vi "Calc Max During Mem Fill 2.vi"(7 "Value":fxp<+/-,22,22>, 8 "LastIterration":bool, 9 "ActiveLedIndex":u32, 10 "FirstIterration":bool, 11 "Address":u32) -> ()   [LabVIEW 2013]
uses:
  <vilib>/rvi/Emulation/niFpgaSctlEmulationGetInTimedLoop.vi
  LIDAR V2 Globals.vi
  <vilib>/rvi/Emulation/niFpgaProcessEmulError.vi
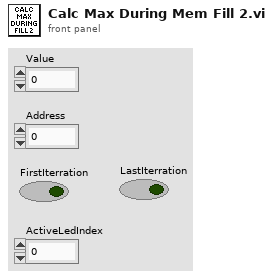
[diagram p1: front panel]
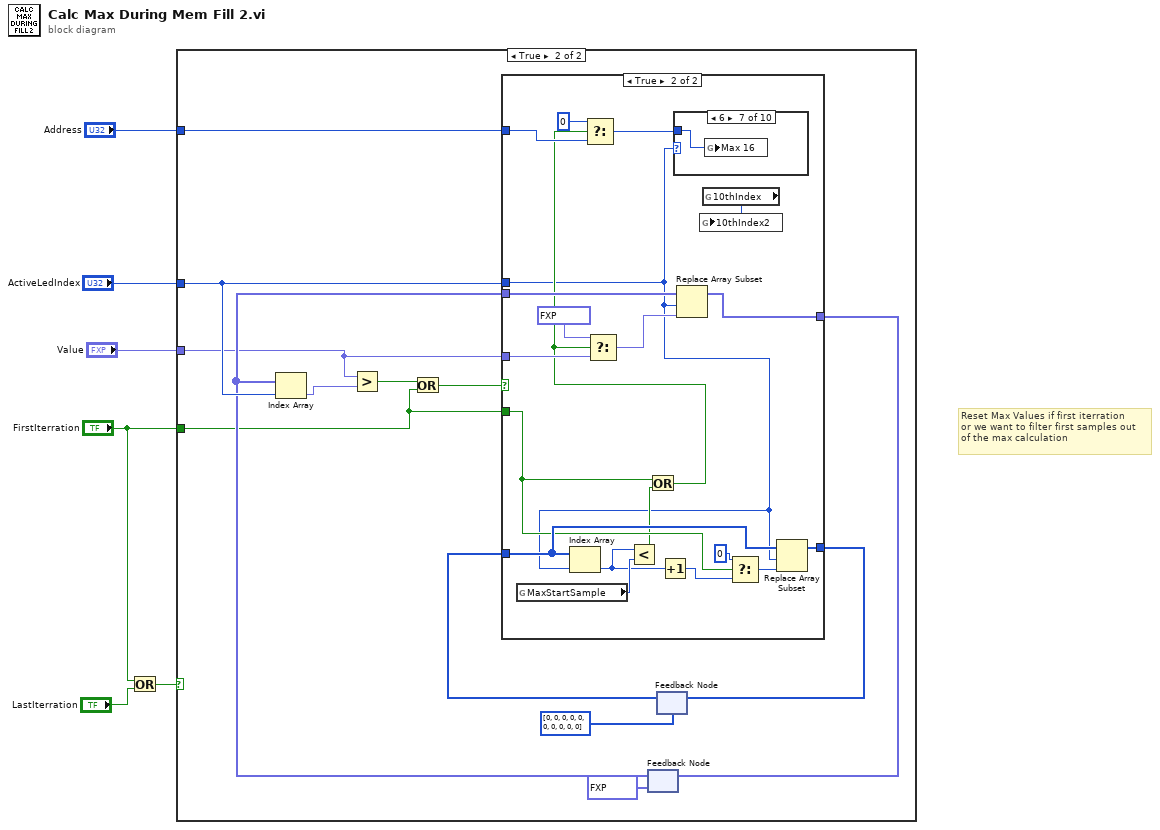
[diagram p0: block diagram]
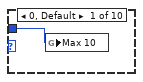
[diagram p4: hidden frame]
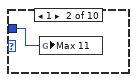
[diagram p5: hidden frame]
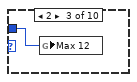
[diagram p6: hidden frame]
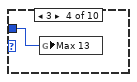
[diagram p7: hidden frame]
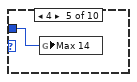
[diagram p8: hidden frame]
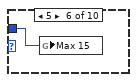
[diagram p9: hidden frame]
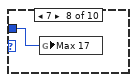
[diagram p10: hidden frame]
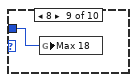
[diagram p11: hidden frame]
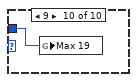
[diagram p12: hidden frame]
diagram:
  # "Reset Max Values if first iterration\nor we want to filter first samples out\nof the max calculation"
  n1 = Or(x="FirstIterration", y="LastIterration") -> (x .or. y?=w1:bool)
  n2 = case shown="True" w1 {
    tunnel: "Address" -> [_ w19]
    tunnel: "ActiveLedIndex" -> [_ w18]
    tunnel: "Value" -> [_ w11]
    tunnel: "FirstIterration" -> [_ w10]
    frame False {
    }
    frame True {
      n3 = feedback #1(fxp<+/-,22,22>[] [0.0, 0.0, 0.0, 0.0, 0.0, 0.0, 0.0, 0.0, 0.0, 0.0]) -> (w14:fxp<+/-,22,22>[])
      n4 = Index Array(array=w14, index=w18) -> (element=w16:fxp<+/-,22,22>)
      n5 = Greater?(x=w11, y=w16) -> (0:w17:bool)
      n6 = Or(x=w17, y=w10) -> (x .or. y?=w13:bool)
      n7 = feedback #2(u8[] [0, 0, 0, 0, 0, 0, 0, 0, 0, 0]) -> (w8:u8[])
      n8 = case shown="True" w13 {
        tunnel: w14 -> [w21 w41]
        tunnel: w11 -> [_ w38]
        tunnel: w18 -> [_ w22]
        tunnel: w19 -> [_ w35]
        tunnel: [w21 w40] -> w15
        tunnel: w10 -> [_ w25]
        tunnel: w8 -> [w20 w27]
        tunnel: [w20 w26] -> w7
        frame False {
        }
        frame True {
          n9 = global read "LIDAR V2 Globals.vi" "MaxStartSample"() -> (w32:u8)
          n10 = Index Array(array=w27, index=w22) -> (element=w31:u8)
          n11 = Less?(x=w31, y=w32) -> (x < y?=w24:bool)
          n12 = Or ("ResetMaxValue")(x=w25, y=w24) -> (x .or. y?=w23:bool)
          n13 = Select(t=u32 0, s=w23, f=w35) -> (s? t:f=w34:u32)
          n14 = Select(t=fxp<+/-,22,22> -2097152.0, s=w23, f=w38) -> (s? t:f=w37:fxp<+/-,22,22>)
          n15 = Increment(x=w31) -> (x+1=w28:u8)
          n16 = case shown="6" w22 {
            tunnel: w34 -> [w42 w43 w44 w45 w46 w47 w48 w49 w50 w51]
            frame 0, Default {
              n17 = global write "LIDAR V2 Globals.vi" "Max 10"(w42) -> ()
            }
            frame 1 {
              n18 = global write "LIDAR V2 Globals.vi" "Max 11"(w43) -> ()
            }
            frame 2 {
              n19 = global write "LIDAR V2 Globals.vi" "Max 12"(w44) -> ()
            }
            frame 3 {
              n20 = global write "LIDAR V2 Globals.vi" "Max 13"(w45) -> ()
            }
            frame 4 {
              n21 = global write "LIDAR V2 Globals.vi" "Max 14"(w46) -> ()
            }
            frame 5 {
              n22 = global write "LIDAR V2 Globals.vi" "Max 15"(w47) -> ()
            }
            frame 6 {
              n23 = global write "LIDAR V2 Globals.vi" "Max 16"(w48) -> ()
            }
            frame 7 {
              n24 = global write "LIDAR V2 Globals.vi" "Max 17"(w49) -> ()
            }
            frame 8 {
              n25 = global write "LIDAR V2 Globals.vi" "Max 18"(w50) -> ()
            }
            frame 9 {
              n26 = global write "LIDAR V2 Globals.vi" "Max 19"(w51) -> ()
            }
          }
          n27 = Replace Array Subset(array=w41, new element=w37, index=w22) -> (w40:fxp<+/-,22,22>[])
          n28 = global read "LIDAR V2 Globals.vi" "10thIndex"() -> (w33:u8)
          n29 = global write "LIDAR V2 Globals.vi" "10thIndex2"(w33) -> ()
          n30 = Select(t=u8 0, s=w25, f=w28) -> (s? t:f=w29:u8)
          n31 = Replace Array Subset(array=w27, new element=w29, index=w22) -> (w26:u8[])
        }
      }
      n32 = feedback-in #1(w15) -> ()
      n33 = feedback-in #2(w7) -> ()
    }
  }
